vi "Scrolling Gradient Color Ramp.vi"() -> ()   [LabVIEW 2010]
panel:
  in  "Clear Colors":bool
  in  "Color Array":u32[](array[colorbox])=[0, 16448250, 0]
  in  "Update":bool
  in  "Speed":u32(knob)=39 scale=0.0..50.0
  in  "stop":bool
  out "1 Pix H - Color Box Array":u32[](array[colorbox])=[14277081, 14145495, 13948116, 13816530, 13619151, 13487565, 13290186, 13092807, 12961221, 12763842, 12632256, 12434877, 12303291, 12105912, 11974326, 11776947, 11645361, 11447982, 11316396, 11119017, 10987431, 10790052, 10658466, 10461087, 10329501, 10132122, 10000536, 9803157, 9605778, 9474192, 9276813, 9145227, 8947848, 8816262, 8618883, 8487297, 8289918, 8158332, 7960953, 7829367, 7631988, 7500402, 7303023, 7171437, 6974058, 6842472, 6645093, 6447714, 6316128, 6118749, 5987163, 5789784, 5658198, 5460819, 5329233, 5131854, 5000268, 4802889, 4671303, 4473924, 4342338, 4144959, 4013373, 3815994, 3684408, 3487029, 3355443, 3158064, 2960685, 2829099, 2631720, 2500134, 2302755, 2171169, 1973790, 1842204, 1644825, 1513239, 1315860, 1184274, 986895, 855309, 657930, 526344, 328965, 197379, 0, 0, 197379, 328965, 526344, 657930, 855309, 986895, 1184274, 1315860, 1513239, 1644825, 1842204, 1973790, 2171169, 2302755, 2500134, 2631720, 2829099, 2960685, 3158064, 3355443, 3487029, 3684408, 3815994, 4013373, 4144959, 4342338, 4473924, 4671303, 4802889, 5000268, 5131854, 5329233, 5460819, 5658198, 5789784, 5987163, 6118749, 6316128, 6447714, 6645093, 6842472, 6974058, 7171437, 7303023, 7500402, 7631988, 7829367, 7960953, 8158332, 8289918, 8487297, 8618883, 8816262, 8947848, 9145227, 9276813, 9474192, 9605778, 9803157, 10000536, 10132122, 10329501, 10461087, 10658466, 10790052, 10987431, 11119017, 11316396, 11447982, 11645361, 11776947, 11974326, 12105912, 12303291, 12434877, 12632256, 12763842, 12961221, 13092807, 13290186, 13487565, 13619151, 13816530, 13948116, 14145495, 14277081, 14474460, 14606046, 14803425, 14935011, 15132390, 15263976, 15461355, 15592941, 15790320, 15921906, 16119285, 16250871, 16448250, 16448250, 16250871, 16119285, 15921906, 15790320, 15592941, 15461355, 15263976, 15132390, 14935011, 14803425, 14606046, 14474460]
  out "1 Pix W - Color Box Array":u32[](array[colorbox])=[14277081, 14145495, 13948116, 13816530, 13619151, 13487565, 13290186, 13092807, 12961221, 12763842, 12632256, 12434877, 12303291, 12105912, 11974326, 11776947, 11645361, 11447982, 11316396, 11119017, 10987431, 10790052, 10658466, 10461087, 10329501, 10132122, 10000536, 9803157, 9605778, 9474192, 9276813, 9145227, 8947848, 8816262, 8618883, 8487297, 8289918, 8158332, 7960953, 7829367, 7631988, 7500402, 7303023, 7171437, 6974058, 6842472, 6645093, 6447714, 6316128, 6118749, 5987163, 5789784, 5658198, 5460819, 5329233, 5131854, 5000268, 4802889, 4671303, 4473924, 4342338, 4144959, 4013373, 3815994, 3684408, 3487029, 3355443, 3158064, 2960685, 2829099, 2631720, 2500134, 2302755, 2171169, 1973790, 1842204, 1644825, 1513239, 1315860, 1184274, 986895, 855309, 657930, 526344, 328965, 197379, 0, 0, 197379, 328965, 526344, 657930, 855309, 986895, 1184274, 1315860, 1513239, 1644825, 1842204, 1973790, 2171169, 2302755, 2500134, 2631720, 2829099, 2960685, 3158064, 3355443, 3487029, 3684408, 3815994, 4013373, 4144959, 4342338, 4473924, 4671303, 4802889, 5000268, 5131854, 5329233, 5460819, 5658198, 5789784, 5987163, 6118749, 6316128, 6447714, 6645093, 6842472, 6974058, 7171437, 7303023, 7500402, 7631988, 7829367, 7960953, 8158332, 8289918, 8487297, 8618883, 8816262, 8947848, 9145227, 9276813, 9474192, 9605778, 9803157, 10000536, 10132122, 10329501, 10461087, 10658466, 10790052, 10987431, 11119017, 11316396, 11447982, 11645361, 11776947, 11974326, 12105912, 12303291, 12434877, 12632256, 12763842, 12961221, 13092807, 13290186, 13487565, 13619151, 13816530, 13948116, 14145495, 14277081, 14474460, 14606046, 14803425, 14935011, 15132390, 15263976, 15461355, 15592941, 15790320, 15921906, 16119285, 16250871, 16448250, 16448250, 16250871, 16119285, 15921906, 15790320, 15592941, 15461355, 15263976, 15132390, 14935011, 14803425, 14606046, 14474460]
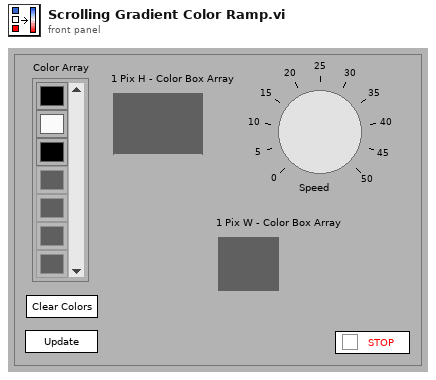
[diagram p1: front panel]
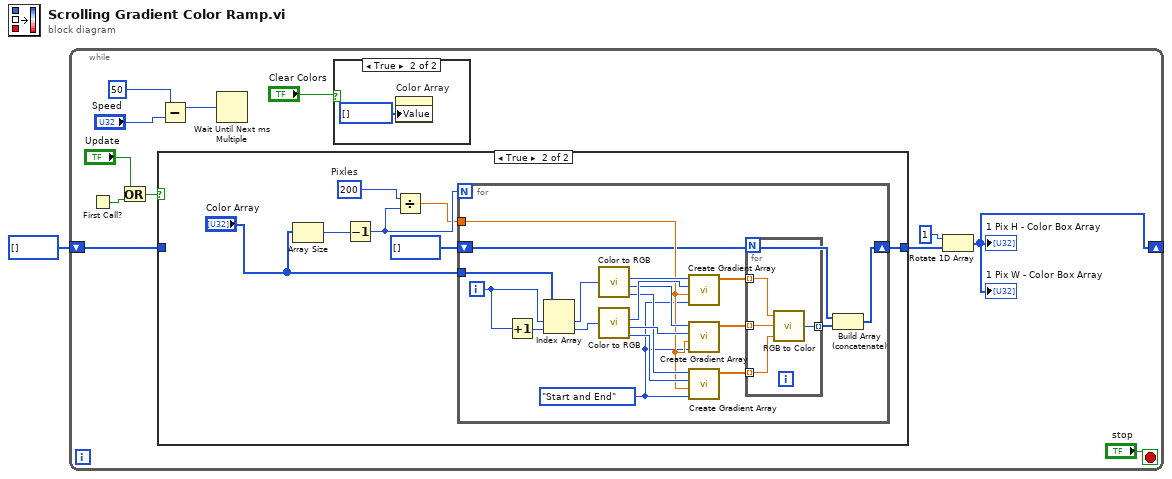
[diagram p0: block diagram]
diagram:
  n1 = while {
    shift-right: [w12] -> _
    shift-left: u32[] [] -> [w6]
    stop <- "stop" stop-if-true
    n2 = First Call?() -> (First Call?: T/F=w9:bool)
    n3 = Or(x="Update", y=w9) -> (x .or. y?=w8:bool)
    n4 = case shown="True" w8 {
      tunnel: [w15 w17] -> w7
      tunnel: w6 -> [w15 _]
      frame False {
      }
      frame True {
        w18 = 200  # Pixles
        n5 = Array Size(array="Color Array") -> (size(s)=w21:i32)
        n6 = Decrement(x=w21) -> (x-1=w22:i32)
        n7 = Divide(x=w18, y=w22) -> (x/y=w19:dbl)
        n8 = for {
          N: w22 -> [_]
          tunnel: "Color Array" -> [w41]
          tunnel: w19 -> [w30]
          shift-right: [w23] -> w17
          shift-left: u32[] [] -> [w24]
          i -> [w40]
          w29 = enum16{"Start", "End", "Start and End", "None"}."Start and End" ("Values to Include")
          n9 = Increment(x=w40) -> (x+1=w39:i32)
          n10 = Index Array(array=w41, index #1=w40, index #2=w39) -> (element #1=w38:u32, element #2=w37:u32)
          n11 = call <vilib>:"Color to RGB.vi"("Color"=w38) -> ("R"=w36:u8, "G"=w34:u8, "B"=w32:u8)  [unwired: 1 out]
          n12 = call <vilib>:"Color to RGB.vi"("Color"=w37) -> ("R"=w35:u8, "G"=w33:u8, "B"=w31:u8)  [unwired: 1 out]
          n13 = call "Create Gradient Array.vi"("Values to Include"=w29, "Array Length"=w30, "End Value"=w35, "Start Value"=w36) -> ("Output Array"=w28:dbl[])  [unwired: 7 in]
          n14 = call "Create Gradient Array.vi"("Values to Include"=w29, "Array Length"=w30, "End Value"=w33, "Start Value"=w34) -> ("Output Array"=w27:dbl[])  [unwired: 7 in]
          n15 = call "Create Gradient Array.vi"("Values to Include"=w29, "Array Length"=w30, "End Value"=w31, "Start Value"=w32) -> ("Output Array"=w26:dbl[])  [unwired: 7 in]
          n16 = for {
            tunnel: w28 -> [w44] mode=indexing
            tunnel: w27 -> [w45] mode=indexing
            tunnel: w26 -> [w43] mode=indexing
            tunnel: [w42] -> w25 mode=indexing
            n17 = call <vilib>:"RGB to Color.vi"("B"=w43, "G"=w45, "R"=w44) -> ("Color"=w42:u32)
          }
          n18 = Build Array (concatenate)(w24, w25) -> (w23:u32[])
        }
      }
    }
    n19 = Subtract(x=u32 50 ("y"), y="Speed") -> (x-y=w3:u32)
    n20 = Wait Until Next ms Multiple(millisecond multiple=w3) -> ()  [unwired: 1 out]
    n21 = case shown="True" "Clear Colors" {
      frame False {
      }
      frame True {
        n22 = property on="Color Array" class="Arr (strict)"("Value"=u32[] [] ("Color Array")) -> ()  [unwired: 2 in, 2 out]
      }
    }
    n23 = Rotate 1D Array(1:w7, 2:1 ("n")) -> (0:w12:u32[])
    "1 Pix H - Color Box Array" <- w12
    "1 Pix W - Color Box Array" <- w12
  }
